vi "Clamp.vi"() -> ()   [LabVIEW 2014]
uses:
  Precreated VIs/Robot Global Data.vi
panel:
  in  "In or Out?":bool
  in  "Limit Max":bool
  in  "Beam Breaker":bool
  in  "Limit Min":bool
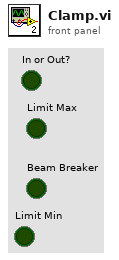
[diagram p1: front panel]
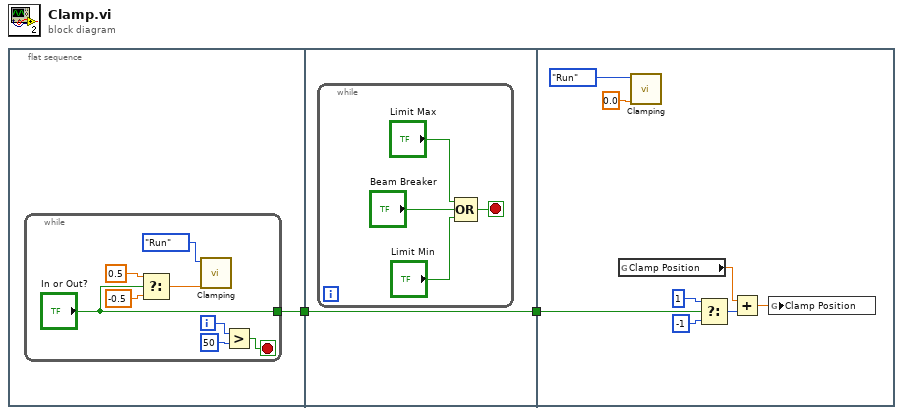
[diagram p0: block diagram]
diagram:
  n1 = flat-sequence {
    tunnel: [w3] -> w1
    tunnel: [w12] -> w2
    tunnel: w1 -> [w12]
    tunnel: w2 -> [w19]
    frame #0 {
      n2 = while {
        tunnel: ["In or Out?"] -> w3
        i -> [w8]
        stop <- w6 stop-if-true
        n3 = Select(t=0.5, s="In or Out?", f=-0.5) -> (s? t:f=w11:dbl)
        n4 = call "Clamping.vi"("Motor Speed"=w11, "Mode"=enum8{"Start", "Run", "Finish"}."Run") -> ()  [unwired: 10 in]
        n5 = Greater?(x=w8, y=50) -> (0:w6:bool)
      }
    }
    frame #1 {
      n6 = while {
        stop <- w16 stop-if-true
        n7 = Compound Arithmetic op=OR("Limit Max", "Beam Breaker", "Limit Min") -> (w16:bool)
      }
    }
    frame #2 {
      n8 = global read "Robot Global Data.vi" "Clamp Position"() -> (w22:dbl)
      n9 = call "Clamping.vi"("Motor Speed"=0.0, "Mode"=enum8{"Start", "Run", "Finish"}."Run") -> ()  [unwired: 10 in]
      n10 = Select(t=1, s=w19, f=-1) -> (s? t:f=w21:i32)
      n11 = Add(x=w22, y=w21) -> (x+y=w20:dbl)
      n12 = global write "Robot Global Data.vi" "Clamp Position"(w20) -> ()
    }
  }
